vi "ReadDataFile_V2.vi"(6 "Channel Name Array Size":i32, 7 "Resolution":string, 8 "error in (no error)":errorcluster, 9 "Create CSV files?":bool, 10 "Channel Name Individual":string, 11 "DataFolder Path":path) -> (0 "error out":errorcluster, 2 "Current Measurements Individual":cluster{dbl[], dbl[]}, 3 "Voltage Measurements Individual":cluster{dbl[], dbl[]})   [LabVIEW 2019]
uses:
  <vilib>/Utility/file.llb/Write Delimited Spreadsheet (string).vi
panel:
  in  "Channel Names Array":string[](array[string])
  out "Voltage Measurements":cluster{dbl[], dbl[]}[](array[cluster])
  out "Current Measurements":cluster{dbl[], dbl[]}[](array[cluster])
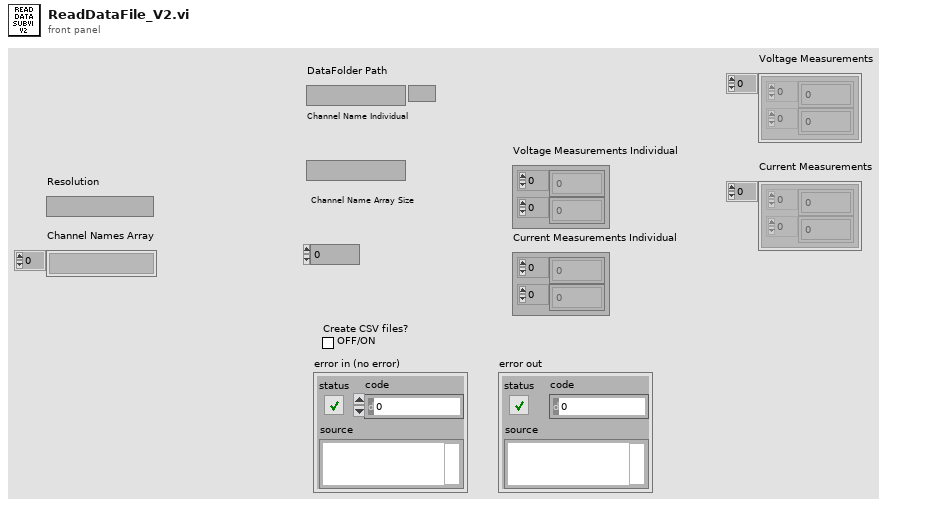
[diagram p1: front panel]
types:
  T1 = enum16{"big-endian, network order", "native, host order", "little-endian"}
  T2 = cluster{"Array of fetched data":dbl[][], string, i32[]}
  T3 = enum16{"open", "replace", "create", "open or create", "replace or create", "replace or create with confirmation"}
  T4 = cluster{"Array of fetched data":dbl[][], string, i32[]}[]
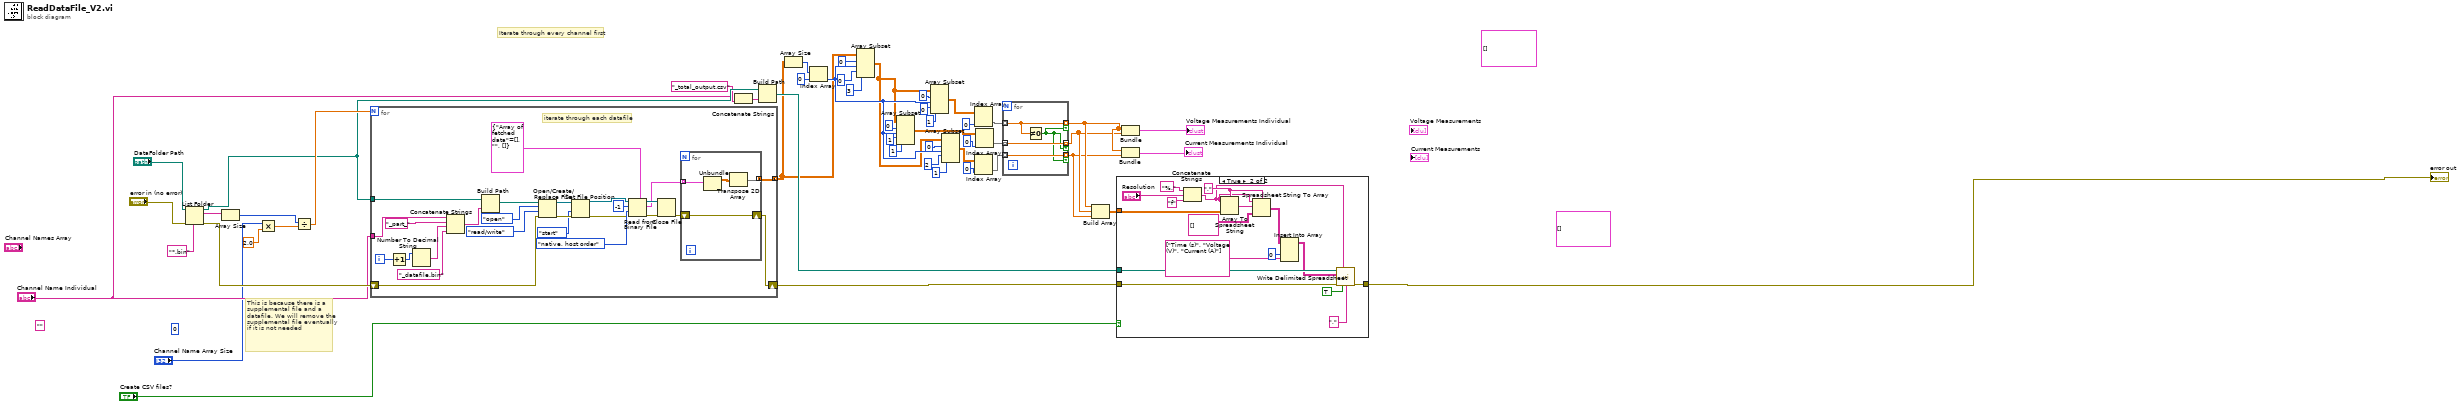
[diagram p0: block diagram]
diagram:
  (unwired) 0
  (unwired) ""
  (unwired) cluster{dbl[], dbl[]}[] []
  (unwired) cluster{dbl[], dbl[]}[] []
  # "Iterate through every channel first"
  # "This is because there is a supplemental file and a datafile. We will remove the supplemental file eventually if it is not needed"
  n1 = List Folder(path="DataFolder Path", pattern="*.bin", error in="error in (no error)") -> (path out=w45:path, filenames=w41:string[], error out=w47:errorcluster)  [unwired: 1 in, 1 out]
  n2 = Array Size(array=w41) -> (size(s)=w44:i32)
  n3 = Multiply(x="Channel Name Array Size", y=2.0) -> (x*y=w43:dbl)
  n4 = Divide(x=w44, y=w43) -> (x/y=w46:dbl)
  n5 = for {
    N: w46 -> [_]
    tunnel: "Channel Name Individual" -> [w76]
    tunnel: w45 -> [w72]
    shift-right: [w52] -> w33
    shift-left: w47 -> [w67]
    tunnel: [w51] -> w10 mode=concatenating
    i -> [w56]
    # "iterate through each datafile"
    n6 = Increment(x=w56) -> (x+1=w55:i32)
    n7 = Number To Decimal String(number=w55) -> (decimal integer string=w74:string)  [unwired: 1 in]
    n8 = Concatenate Strings(w76, "_part_" ("string"), w74, "_datafile.bin" ("string")) -> (w71:string)
    n9 = Build Path(base path=w72, name or relative path=w71) -> (appended path=w70:path)
    n10 = Open/Create/Replace File(file path (use dialog)=w70, error in=w67, operation (0:open)=T3."open", access (0:read/write)=enum16{"read/write", "read-only", "write-only"}."read/write") -> (refnum out=w60:refnum<file>, error out=w61:errorcluster)  [unwired: 2 in, 1 out]
    n11 = Set File Position(refnum=w60, from (0:start)=enum16{"start", "end", "current"}."start", error in=w61) -> (refnum out=w57:refnum<file>, error out=w58:errorcluster)  [unwired: 1 in]
    n12 = Read from Binary File(5:T2 {"Array of fetched data"=[], "", []} ("cluster"), 8:w58, 9:T1."native, host order" ("byte order (0:big-endian, network order)"), 10:-1 ("count (1)"), 11:w57) -> (0:w63:errorcluster, 2:w54:T4, 3:w62:refnum<file>)  [unwired: 1 in, 1 out]
    n13 = Close File(refnum=w62, error in=w63) -> (error out=w53:errorcluster)  [unwired: 1 out]
    n14 = for {
      tunnel: w54 -> [w80] mode=indexing
      tunnel: [w77] -> w51 mode=concatenating
      shift-right: [w79] -> w52
      shift-left: w53 -> [w79]
      n15 = Unbundle(w80) -> ("Array of fetched data"=w78:dbl[][])  [unwired: 2 out]
      n16 = Transpose 2D Array(2D array=w78) -> (transposed array=w77:dbl[][])
    }
  }
  n17 = Concatenate Strings("Channel Name Individual", "_total_output.csv" ("string")) -> (w36:string)
  n18 = Build Path(base path=w45, name or relative path=w36) -> (appended path=w34:path)
  n19 = Array Size(array=w10) -> (size(s)=w38:i32[])
  n20 = Index Array(array=w38, index=0) -> (element=w20:i32)
  n21 = Array Subset(array=w10, index (row)=0 ("index"), length (row)=w20, index (col)=0 ("index"), length (col)=3 ("length")) -> (w9:dbl[][])
  n22 = Array Subset(array=w9, index (row)=0 ("index"), length (row)=w20, index (col)=1 ("index"), length (col)=1 ("length")) -> (w18:dbl[][])
  n23 = Array Subset(array=w9, index (row)=0 ("index"), length (row)=w20, index (col)=0 ("index"), length (col)=1 ("length")) -> (w19:dbl[][])
  n24 = Array Subset(array=w9, index (row)=0 ("index"), length (row)=w20, index (col)=2 ("index"), length (col)=1 ("length")) -> (w17:dbl[][])
  n25 = Index Array(array=w19, index (col)=0 ("disabled index (col)")) -> (element=w13:dbl[])  [unwired: 1 in]
  n26 = Index Array(array=w17, index (col)=0 ("disabled index (col)")) -> (element=w11:dbl[])  [unwired: 1 in]
  n27 = Index Array(array=w18, index (col)=0 ("disabled index (col)")) -> (element=w12:dbl[])  [unwired: 1 in]
  n28 = for {
    tunnel: w13 -> [w81] mode=indexing
    tunnel: w12 -> [w84] mode=indexing
    tunnel: w11 -> [w83] mode=indexing
    tunnel: [w81] -> w8 mode=indexing if=w82
    tunnel: [w84] -> w7 mode=indexing if=w82
    tunnel: [w83] -> w6 mode=indexing if=w82
    n29 = Not Equal To 0?(x=w81) -> (x != 0?=w82:bool)
  }
  n30 = Build Array(w8, w7, w6) -> (w5:dbl[][])
  n31 = case shown="True" "Create CSV files?" {
    tunnel: w34 -> [_ w102]
    tunnel: w33 -> [w85 w101]
    tunnel: [w85 w100] -> w39
    tunnel: w5 -> [_ w94]
    frame False {
    }
    frame True {
      w98 = "," ("delimiter (Tab)")
      n32 = Concatenate Strings("%." ("string"), "Resolution", "f" ("string")) -> (w87:string)
      n33 = Array To Spreadsheet String(delimiter (Tab)=w98, array=w94, 3:w87) -> (spreadsheet string=w97:string)
      n34 = Spreadsheet String To Array(delimiter (Tab)=w98, format string=w87, spreadsheet string=w97, array type (2D Dbl)=string[][] []) -> (array=w93:string[][])
      n35 = Insert Into Array(array=w93, index (col)=0 ("disabled index (col)"), new element=string[] ["Time (s)", "Voltage (V)", "Current (A)"]) -> (w91:string[][])  [unwired: 1 in]
      n36 = call-poly <vilib>:"Write Delimited Spreadsheet.vi"("file path (dialog if empty)"=w102, "format (%s)"=w87, "2D data"=w91, "error in (no error)"=w101, "transpose? (no:F)"=TRUE, "delimiter (\\t)"="," ("delimiter (\\t)")) -> ("error out"=w100:errorcluster)  [unwired: 8 in, 1 out]
    }
  }
  "error out" <- w39
  n37 = Bundle(w8, w6) -> (→"Current Measurements Individual":cluster{dbl[], dbl[]})  [unwired: 1 in]
  n38 = Bundle(w8, w7) -> (→"Voltage Measurements Individual":cluster{dbl[], dbl[]})  [unwired: 1 in]
